vi "DSF.Engine.Framework.Get Engine Channels Pointer.vi"(11 "Framework in":refnum<class "DSF.Engine.Framework.lvclass">) -> (2 "Engine Channels Pointer":refnum<class "DSF.Engine.Pointer.DBL.lvclass">, 3 "Framework out":refnum<class "DSF.Engine.Framework.lvclass">)   [LabVIEW 2017, in "DSF.Engine.lvlib" / "DSF.Engine.Framework.lvclass"]
uses:
  DSF.Engine.Framework.lvclass
  Pointer/DSF.Engine.Pointer.DBL.lvclass
  DSF.Engine.Framework.lvclass/DSF.Engine.Framework.ctl
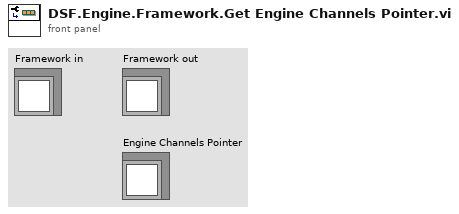
[diagram p1: front panel]
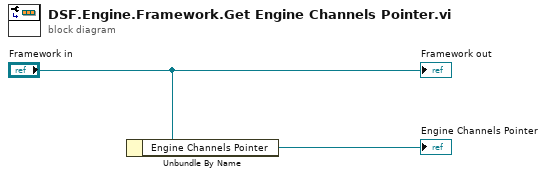
[diagram p0: block diagram]
diagram:
  n1 = Unbundle By Name("Framework in") -> ("Engine Channels Pointer"=→"Engine Channels Pointer":refnum<class "DSF.Engine.Pointer.DBL.lvclass">)
  "Framework out" <- "Framework in"
